vi "Segmented Averager Test.vi"() -> ()   [LabVIEW 2018]
uses:
  56269e73-51c6-4221-8fb7-e2d3707ba361.vi
  56269e73-51c6-4221-8fb7-e2d3707ba361.vi/e2d8b3ab-e410-40e6-b680-0b91d3120afd.vi
panel:
  out "P-P":dbl[](array[numeric])
  out "Average":dbl
  out "Array Out":dbl[][](array[numeric])
  out "Array In":dbl[](array[numeric])
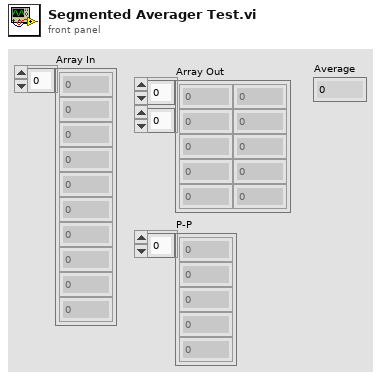
[diagram p1: front panel]
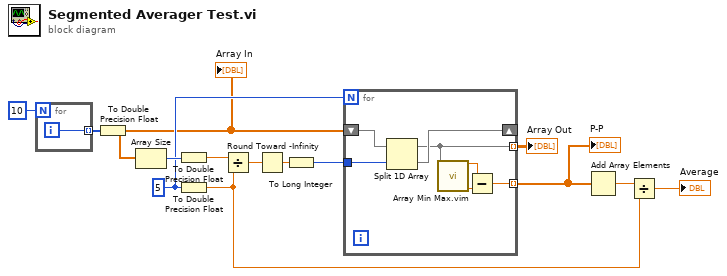
[diagram p0: block diagram]
diagram:
  w7 = 5 ("number")
  n1 = for {
    N: 10 -> [_]
    tunnel: [w15] -> w13 mode=indexing
    i -> [w15]
  }
  n2 = To Double Precision Float(number=w13) -> (double precision float=w6:dbl[])
  "Array In" <- w6
  n3 = Array Size(array=w6) -> (size(s)=w11:i32)
  n4 = To Double Precision Float(number=w11) -> (double precision float=w9:dbl)
  n5 = To Double Precision Float(number=w7) -> (double precision float=w2:dbl)
  n6 = Divide(x=w9, y=w2) -> (x/y=w10:dbl)
  n7 = Round Toward -Infinity(1:w10) -> (0:w12:dbl)
  n8 = To Long Integer(number=w12) -> (32bit integer=w8:i32)
  n9 = for {
    N: w7 -> [_]
    tunnel: w8 -> [w20]
    shift-right: [w21] -> _
    shift-left: w6 -> [w22]
    tunnel: [w19] -> w5 mode=indexing
    tunnel: [w16] -> w4 mode=indexing
    n10 = Split 1D Array(array=w22, index=w20) -> (first subarray=w19:dbl[], second subarray=w21:dbl[])
    n11 = call "Array Min Max.vim"("Array"=w19) -> ("Max"=w18:dbl, "Min"=w17:dbl)  [unwired: 13 in]
    n12 = Subtract(x=w18, y=w17) -> (x-y=w16:dbl)
  }
  "Array Out" <- w5
  "P-P" <- w4
  n13 = Add Array Elements(numeric array=w4) -> (sum=w3:dbl)
  n14 = Divide(x=w3, y=w2) -> (x/y=→"Average":dbl)
